vi "Motion.vi"(9 "engine start":bool, 10 "coerced":dbl, 11 "BRAKES":bool) -> (3 "upper limit":dbl)   [LabVIEW 2015]
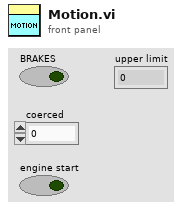
[diagram p1: front panel]
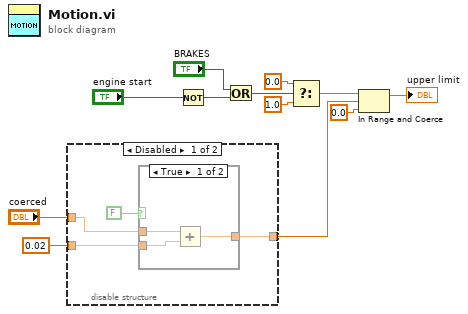
[diagram p0: block diagram]
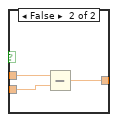
[diagram p2: hidden frame]
diagram:
  n1 = disable-structure shown="Disabled" {
    disable-tunnel: 0.02 -> [w16 _]
    disable-tunnel: [w15 w23] -> w3
    disable-tunnel: "coerced" -> [w14 w23]
    frame Disabled {
      n2 = case shown="True" FALSE {
        tunnel: w14 -> [w18 w22]
        tunnel: w16 -> [w19 w20]
        tunnel: [w17 w21] -> w15
        frame True {
          n3 = Add(x=w18, y=w19) -> (x+y=w17:dbl)
        }
        frame False {
          n4 = Subtract(x=w22, y=w20) -> (x-y=w21:dbl)
        }
      }
    }
    frame Enabled {
    }
  }
  n5 = Not(x="engine start") -> (.not. x?=w11:bool)
  n6 = Or(x="BRAKES", y=w11) -> (x .or. y?=w9:bool)
  n7 = Select(t=0.0, s=w9, f=1.0 ("upper limit")) -> (s? t:f=w8:dbl)
  n8 = In Range and Coerce(upper limit=w8, x=w3, lower limit=0.0) -> (coerced(x)=→"upper limit":dbl)  [unwired: 1 out]
